vi "RotateArrayCCW.vi"(1 "Units":enum16{"mrad", "Radians", "Degrees"}(ring)=enum."Radians", 2 "Angle":dbl, 3 "X, Y, Z Input":dbl[](array[numeric]) format="%#_13g") -> (0 "X', Y', Z Output":dbl[](array[numeric]))   [LabVIEW 2016]
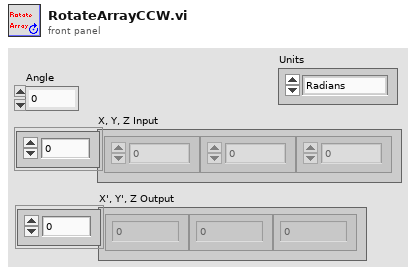
[diagram p1: front panel]
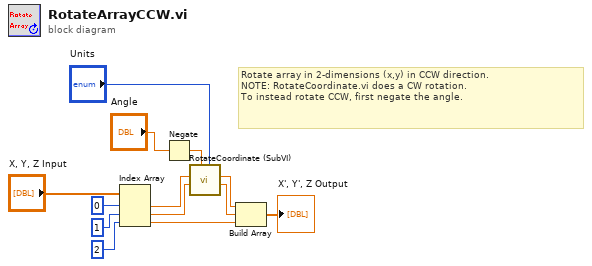
[diagram p0: block diagram]
diagram:
  # "Rotate array in 2-dimensions (x,y) in CCW direction.\nNOTE: RotateCoordinate.vi does a CW rotation.\nTo instead rotate CCW, first negate the angle."
  n1 = Index Array(array="X, Y, Z Input", index #1=0 ("index"), index #2=1 ("index"), index #3=2 ("index")) -> (element #1=w11:dbl, element #2=w12:dbl, element #3=w3:dbl)
  n2 = Negate(x="Angle") -> (-x=w1:dbl)
  n3 = call "RotateCoordinate (SubVI).vi"("Units"="Units", "Angle"=w1, "y"=w12, "x"=w11) -> ("y'"=w6:dbl, "x'"=w7:dbl)  [unwired: 5 in, 1 out]
  n4 = Build Array(w7, w6, w3) -> (→"X', Y', Z Output":dbl[])
